vi "Can File be in LLB.vi"(8 "error in (no error)":errorcluster, 11 "path":path) -> (0 "error out":errorcluster, 3 "Can be in LLB?":bool)   [LabVIEW 2019, in "NI_FileType.lvlib"]
doc: "Returns TRUE if this file could be copied into an LLB."
uses:
  NI_FileType.lvlib
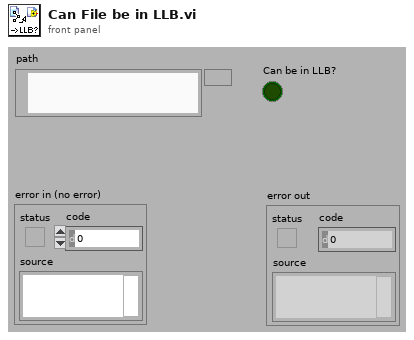
[diagram p1: front panel]
types:
  T1 = typedef "NI_FileType.lvlib/FT_FileTypes.ctl" = enum32{"Invalid file/path", "Unknown type", "Instrument", "Control", "Polymorphic VI", "Project", "Library", "LVClass", "XControl", "XNode", "CIN", "Run-time menu", "Palette menu", "LLB", "Shortcut", "Directory", "Class Private Data Control", "Statechart", "MathScript .m file", "Ladder Diagram", "LVLibp"}
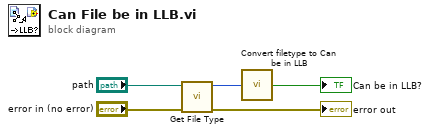
[diagram p0: block diagram]
diagram:
  n1 = call "Get File Type.vi"("error in (no error)"="error in (no error)", "path"="path") -> ("error out"=→"error out":errorcluster, "file type"=w2:T1)  [unwired: 7 in, 1 out]
  n2 = call "Convert filetype to Can be in LLB.vi"("file type"=w2) -> ("Can be in LLB?"=→"Can be in LLB?":bool)  [unwired: 4 in]
